vi "DevconUtil.vi"(6 "error in (no error)":errorcluster, 8 "COM":string, 9 "Action":string(combo)="status") -> (0 "error out":errorcluster, 2 "Standard Output":string="USB\\VID_05E0&PID_1701\\USB_CDC_SYMBOL_SCANNER\r\n    Name: Motorola Scanner Virtual USB COM Port (COM10)\r\n    Driver is running.\r\n1 matching device(s) found.\r\n", 3 "success?":bool)   [LabVIEW 2014]
uses:
  <vilib>/addons/TestStand/_TSLegacy.llb/LabVIEW Test - Test Data.ctl
panel:
  out "Test Data":T1={"PASS/FAIL Flag"=FALSE, "Numeric Measurement"=0.0, "String Measurement"="", "Report Text"="USB\\VID_05E0&PID_1701\\USB_CDC_SYMBOL_SCANNER\r\n    Name: Motorola Scanner Virtual USB COM Port (COM10)\r\n    Driver is running.\r\n1 matching device(s) found.\r\n"} {"Numeric Measurement" format="%.2f"}
  in  "?":path=path "C:/WINDOWS/devcon.exe"
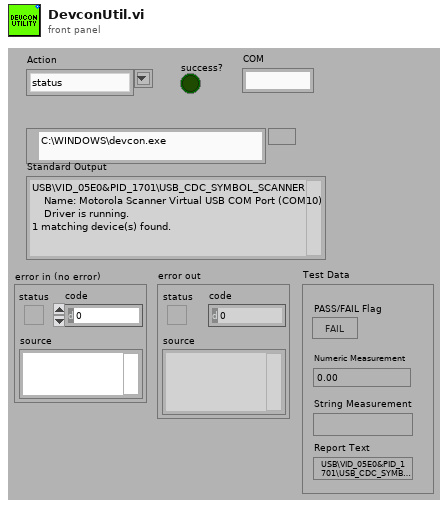
[diagram p1: front panel]
types:
  T1 = typedef "LabVIEW Test - Test Data.ctl" = cluster{"PASS/FAIL Flag":bool, "Numeric Measurement":dbl, "String Measurement":string, "Report Text":string}
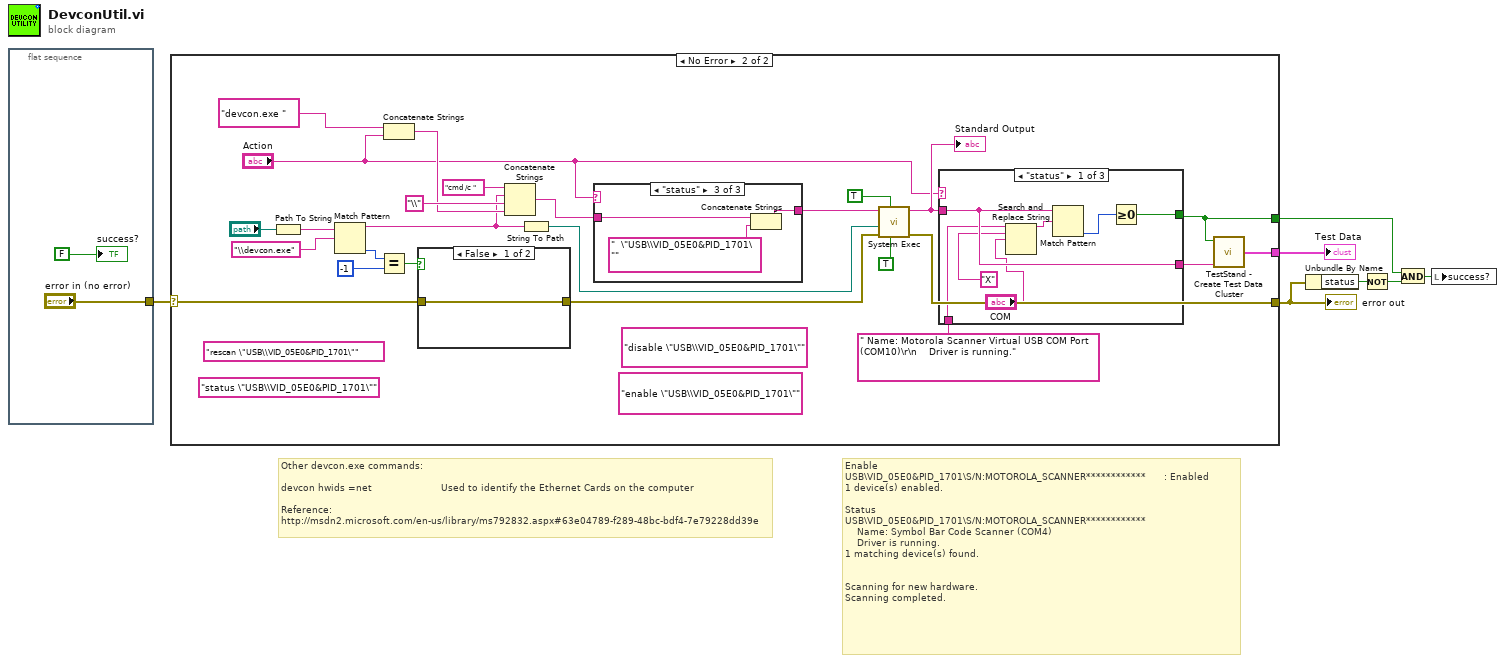
[diagram p0: block diagram]
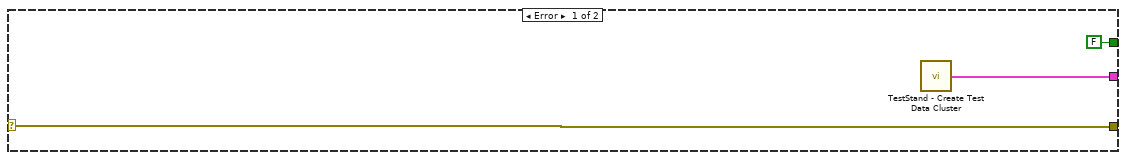
[diagram p2: hidden frame]
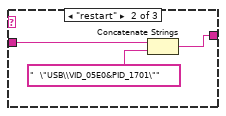
[diagram p4: hidden frame]
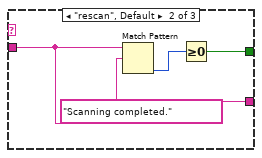
[diagram p5: hidden frame]
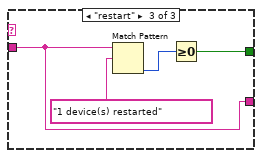
[diagram p6: hidden frame]
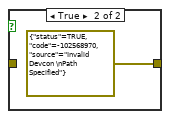
[diagram p7: hidden frame]
diagram:
  # "Enable\nUSB\\VID_05E0&PID_1701\\S/N:MOTOROLA_SCANNER************      : Enabled\n1 device(s) enabled.\n\nStatus\nUSB\\VID_05E0&PID_1701\\S/N:MOTOROLA_SCANNER************\n    Name: Symbol Bar Code Scanner (COM4)\n    Driver is running.\n1 matching device(s) found.\n\n\nScanning for new hardware.\nScanning completed."
  # "Other devcon.exe commands:\n\ndevcon hwids =net                       Used to identify the Ethernet Cards on the computer\n\nReference:\nhttp://msdn2.microsoft.com/en-us/library/ms792832.aspx#63e04789-f289-48bc-bdf4-7e79228dd39e"
  n1 = flat-sequence {
    tunnel: ["error in (no error)"] -> w7
    frame #0 {
      "success?" <- FALSE ("success?")
    }
  }
  n2 = case shown="No Error" w7 {
    selector: w7 -> [w12 w26]
    tunnel: [w12 w22] -> w5
    tunnel: [w11 w23] -> w6
    tunnel: [FALSE w14] -> w2
    frame Error {
      n3 = call <vilib>:"TestStand - Create Test Data Cluster.vi"() -> ("Test Data"=w11:T1)  [unwired: 4 in]
    }
    frame No Error {
      (unwired) "enable \"USB\\VID_05E0&PID_1701\""
      (unwired) "disable \"USB\\VID_05E0&PID_1701\""
      (unwired) "rescan \"USB\\VID_05E0&PID_1701\""
      (unwired) "status \"USB\\VID_05E0&PID_1701\""
      n4 = Path To String(path="?") -> (string=w31:string)
      n5 = Match Pattern(string=w31, regular expression="\\devcon.exe") -> (before substring=w29:string, offset past match=w27:i32)  [unwired: 1 in, 2 out]
      n6 = Equal?(x=w27, y=-1) -> (x = y?=w24:bool)
      n7 = Concatenate Strings("devcon.exe ", "Action") -> (w34:string)
      n8 = case shown="False" w24 {
        tunnel: w26 -> [w60 _]
        tunnel: [w60 errorcluster {"status"=TRUE, "code"=-102568970, "source"="Invalid Devcon \nPath Specified"} ("error IO")] -> w25
        frame False {
        }
        frame True {
        }
      }
      n9 = Concatenate Strings("cmd /c " ("command line"), w29, "\\" ("string"), w34) -> (w18:string)
      n10 = String To Path(string=w29) -> (path=w19:path)
      n11 = case shown="\"status\"" "Action" {
        tunnel: w18 -> [w38 w40 w44]
        tunnel: [w38 w39 w43] -> w17
        frame "rescan", Default {
        }
        frame "restart" {
          n12 = Concatenate Strings(w40, "  \"USB\\VID_05E0&PID_1701\"") -> (w39:string)
        }
        frame "status" {
          n13 = Concatenate Strings(w44, "  \"USB\\VID_05E0&PID_1701\"") -> (w43:string)
        }
      }
      n14 = call <vilib>:"System Exec.vi"("run minimized? (F)"=TRUE, "wait until completion? (T)"=TRUE, "error in (no error)"=w25, "working directory"=w19, "command line"=w17) -> ("error out"=w22:errorcluster, "standard output"=w16:string)  [unwired: 3 in, 2 out]
      "Standard Output" <- w16
      n15 = case shown="\"status\"" "Action" {
        tunnel: [w51 w55 w57] -> w14
        tunnel: [w48 w54 w56] -> w21
        tunnel: w16 -> [w48 w54 w56]
        tunnel: " Name: Motorola Scanner Virtual USB COM Port (COM10)\r\n    Driver is running." -> [w47 _ _]
        frame "status" {
          n16 = Search and Replace String(input string=w47, search string="X", replace string="COM") -> (result string=w49:string)  [unwired: 5 in, 3 out]
          n17 = Match Pattern(string=w48, regular expression=w49) -> (offset past match=w50:i32)  [unwired: 1 in, 3 out]
          n18 = Greater Or Equal To 0?(x=w50) -> (x >= 0?=w51:bool)
        }
        frame "rescan", Default {
          n19 = Match Pattern(string=w54, regular expression="Scanning completed.") -> (offset past match=w53:i32)  [unwired: 1 in, 3 out]
          n20 = Greater Or Equal To 0?(x=w53) -> (x >= 0?=w55:bool)
        }
        frame "restart" {
          n21 = Match Pattern(string=w56, regular expression="1 device(s) restarted") -> (offset past match=w59:i32)  [unwired: 1 in, 3 out]
          n22 = Greater Or Equal To 0?(x=w59) -> (x >= 0?=w57:bool)
        }
      }
      n23 = call <vilib>:"TestStand - Create Test Data Cluster.vi"("Report Text"=w21, "PASS/FAIL Flag"=w14) -> ("Test Data"=w23:T1)  [unwired: 2 in]
    }
  }
  "error out" <- w5
  "Test Data" <- w6
  n24 = Unbundle By Name(w5) -> ("status"=w4:bool)
  n25 = Not(x=w4) -> (.not. x?=w3:bool)
  n26 = And(x=w2, y=w3) -> (x .and. y?=w1:bool)
  n27 = local write "success?"(w1) -> ()
